vi "Table Select Section Paste From 1D Array.vi"(8 "Column Size":i32=-1, 9 "Paste Value":string[](array[string]), 11 "Table Ref In":refnum<vi>) -> (3 "Table Ref Out":refnum<vi>)   [LabVIEW 2024]
uses:
  Converter/String Trimming 2D to 1D.vi
  <vilib>/Utility/miscctls.llb/LVRowAndColumnTypeDef.ctl
panel:
  out "Selection Start":T1
  out "output array":string[][](array[string])
  out "Value":string[][](array[string])
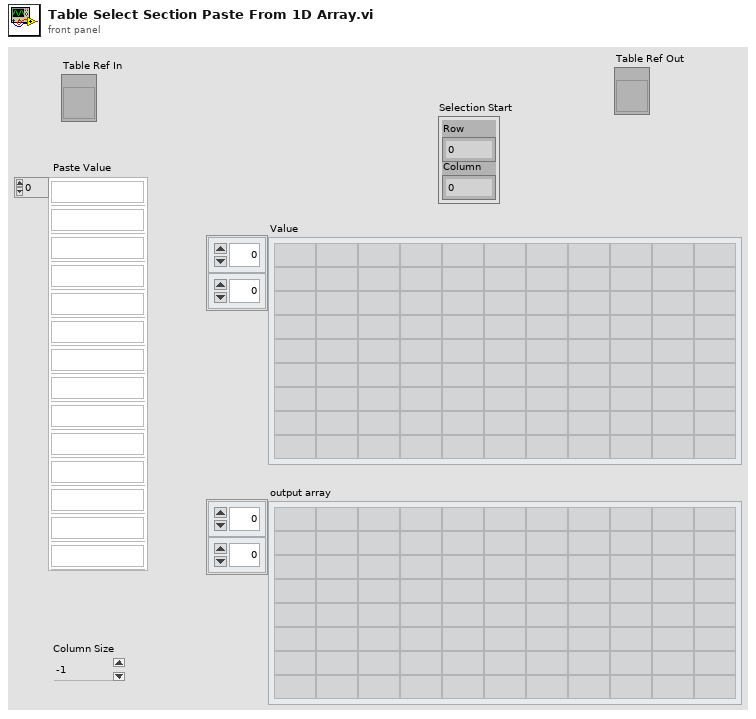
[diagram p1: front panel]
types:
  T1 = typedef "LVRowAndColumnTypeDef.ctl" = cluster{"Row":i32, "Column":i32}
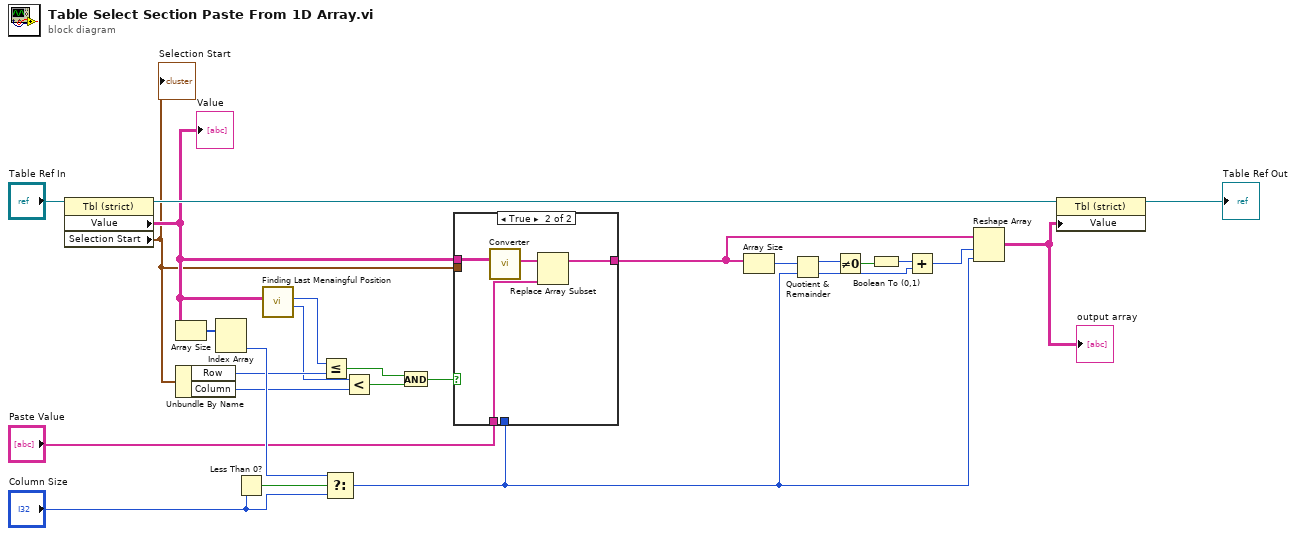
[diagram p0: block diagram]
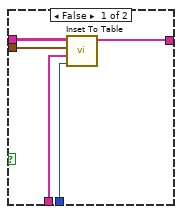
[diagram p2: hidden frame]
diagram:
  n1 = property class="Tbl (strict)"(reference="Table Ref In") -> (reference out=w24:refnum<vi>, "Value"=w10:string[][], "Selection Start"=w1:T1)  [unwired: 1 in, 1 out]
  "Value" <- w10
  "Selection Start" <- w1
  n2 = Array Size(array=w10) -> (size(s)=w23:i32[])
  n3 = Unbundle By Name(w1) -> ("Row"=w9:i32, "Column"=w6:i32)
  n4 = Index Array(array=w23) -> (element #2=w15:i32)  [unwired: 2 in, 1 out]
  n5 = Less Than 0?(x="Column Size") -> (x < 0?=w16:bool)
  n6 = call "Finding Last Menaingful Position.vi"("Data In"=w10) -> ("Column Index"=w7:i32, "Row Index"=w8:i32)  [unwired: 9 in]
  n7 = Less Or Equal?(x=w8, y=w9) -> (x <= y?=w5:bool)
  n8 = Select(t=w15, s=w16, f="Column Size") -> (s? t:f=w2:i32)
  n9 = Less?(x=w7, y=w6) -> (x < y?=w4:bool)
  n10 = And(x=w5, y=w4) -> (x .and. y?=w3:bool)
  n11 = case shown="True" w3 {
    tunnel: w10 -> [w31 w34]
    tunnel: [w30 w33] -> w12
    tunnel: "Paste Value" -> [w29 w32]
    tunnel: w2 -> [w28 _]
    tunnel: w1 -> [w27 _]
    frame False {
      n12 = call "Inset To Table.vi"("Column Size"=w28, "Paste Value"=w29, "Selection Start"=w27, "Table Value"=w31) -> ("1D String Out"=w30:string[])  [unwired: 7 in]
    }
    frame True {
      n13 = call-poly "Converter.vi"("1D String In"=w34) -> ("1D String Out"=w35:string[])  [unwired: 10 in]
      n14 = Replace Array Subset(array=w35, new element=w32) -> (w33:string[])  [unwired: 1 in]
    }
  }
  n15 = Array Size(array=w12) -> (size(s)=w22:i32)
  n16 = Quotient & Remainder(x=w22, y=w2) -> (x-y*floor(x/y)=w21:i32, floor(x/y)=w18:i32)
  n17 = Not Equal To 0?(x=w21) -> (x != 0?=w20:bool)
  n18 = Boolean To (0,1)(Boolean=w20) -> (0, 1=w19:i16)
  n19 = Add(x=w19, y=w18) -> (x+y=w17:i32)
  n20 = Reshape Array(w12, w17, w2) -> (w13:string[][])
  "output array" <- w13
  n21 = property class="Tbl (strict)"(reference=w24, "Value"=w13) -> (reference out=→"Table Ref Out":refnum<vi>)  [unwired: 1 in, 1 out]
